vi "isTraceSaturated.vi"(11 "dX/dt in":dbl[](array[numeric])) -> (1 "Waveform Graph":i32[](graph), 2 "Array 2":i32[](array[numeric]), 3 "saturated":bool)   [LabVIEW 2013]
uses:
  <vilib>/Analysis/NI_AALPro.lvlib
panel:
  out "max value":i32
  out "dX/dt in 2":dbl[](graph)
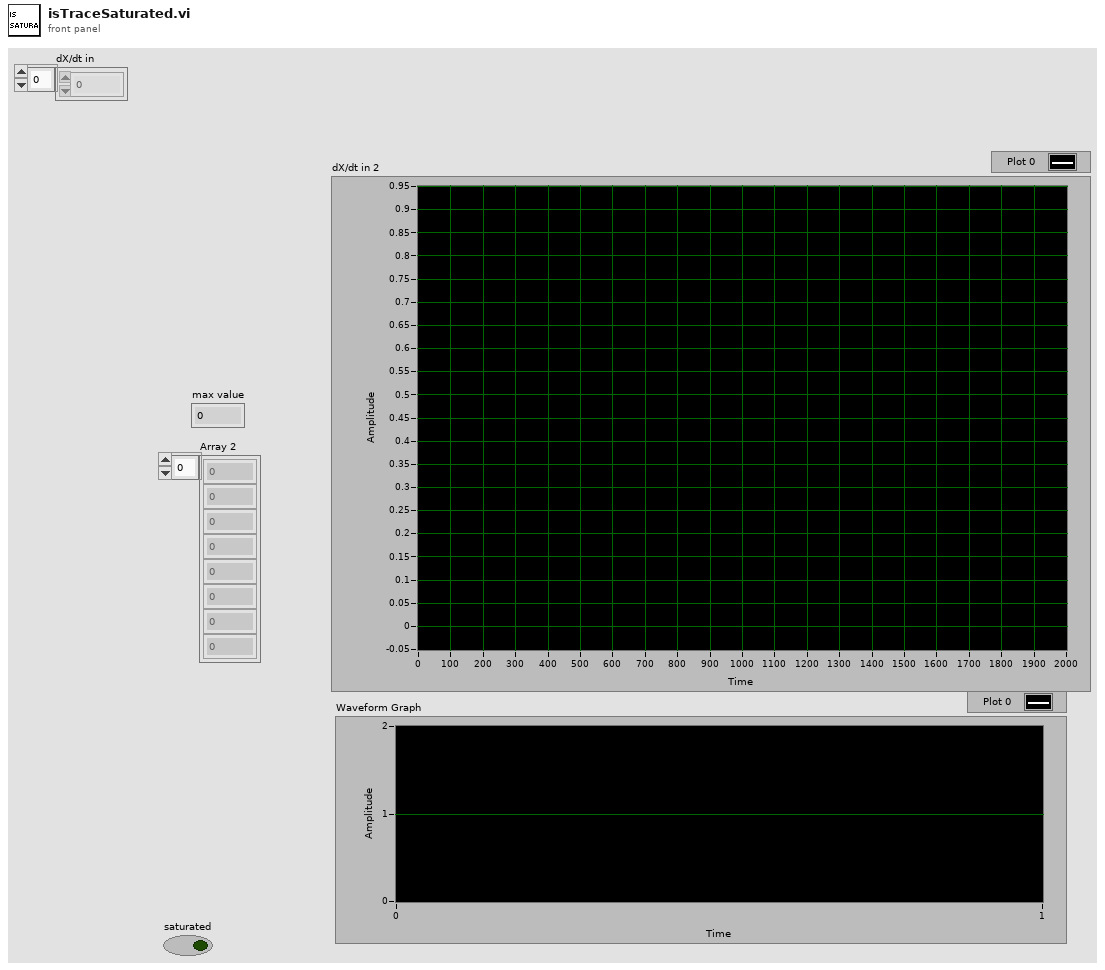
[diagram p1: front panel]
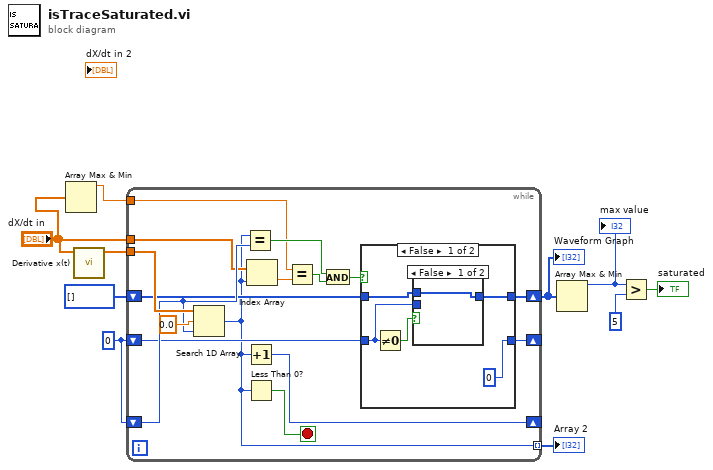
[diagram p0: block diagram]
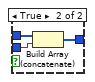
[diagram p2: hidden frame]
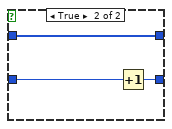
[diagram p3: hidden frame]
diagram:
  w5 = 0
  n1 = Array Max & Min(array="dX/dt in") -> (max value=w1:dbl)  [unwired: 3 out]
  n2 = call <vilib>:"Derivative x(t).vi"("X"="dX/dt in") -> ("dX/dt"=w3:dbl[])  [unwired: 9 in, 1 out]
  n3 = while {
    tunnel: w3 -> [w26]
    shift-right: [w23] -> _
    shift-left: w5 -> [w22]
    tunnel: [w15] -> w4 mode=indexing
    shift-right: [w20] -> _
    shift-left: w5 -> [w21]
    shift-right: [w18] -> w7
    shift-left: i32[] [] -> [w19]
    tunnel: "dX/dt in" -> [w16]
    tunnel: w1 -> [w12]
    stop <- w24 stop-if-true
    n4 = Search 1D Array(1D array=w26, element=0.0, start index (0)=w22) -> (index of element=w15:i32)
    n5 = Equal?(x=w15, y=w22) -> (x = y?=w17:bool)
    n6 = Increment(x=w15) -> (x+1=w23:i32)
    n7 = Less Than 0?(x=w15) -> (x < 0?=w24:bool)
    n8 = Index Array(array=w16, index=w15) -> (element=w13:dbl)
    n9 = Equal?(x=w12, y=w13) -> (x = y?=w11:bool)
    n10 = And(x=w17, y=w11) -> (x .and. y?=w14:bool)
    n11 = case shown="False" w14 {
      tunnel: w21 -> [w28 w38]
      tunnel: [0 w37] -> w20
      tunnel: w19 -> [w30 w36]
      tunnel: [w29 w36] -> w18
      frame False {
        n12 = Not Equal To 0?(x=w28) -> (x != 0?=w27:bool)
        n13 = case shown="False" w27 {
          tunnel: w30 -> [w32 w35]
          tunnel: [w32 w34] -> w29
          tunnel: w28 -> [_ w33]
          frame False {
          }
          frame True {
            n14 = Build Array (concatenate)(w35, w33) -> (w34:i32[])
          }
        }
      }
      frame True {
        n15 = Increment(x=w38) -> (x+1=w37:i32)
      }
    }
  }
  "Array 2" <- w4
  "Waveform Graph" <- w7
  n16 = Array Max & Min(array=w7) -> (max value=w8:i32)  [unwired: 3 out]
  "max value" <- w8
  n17 = Greater?(x=w8, y=5) -> (0:→"saturated":bool)
